vi "Discovery Loop Async.vi"(11 "DiscoveryService in":refnum<class "DiscoveryService.lvclass">) -> ()   [LabVIEW 2020, in "Vecto.lvlib" / "DiscoveryService.lvclass"]
uses:
  DiscoveryService.lvclass
  DiscoveryService.lvclass/DiscoveryService.ctl
  lv-volatus/messages/Discovery/Class/Msg.lvclass
  lv-volatus/messages/ServiceType/Enumeration.ctl
  lv-volatus/messages/ServiceType/ServiceType.lvlib
  lv-volatus/messages/Service/Data.ctl
  lv-volatus/messages/Service/Service.lvlib
  lv-volatus/messages/Discovery/Data.ctl
  lv-volatus/messages/Discovery/Discovery.lvlib
panel:
  out "Nodes":T1[](array[typedef])
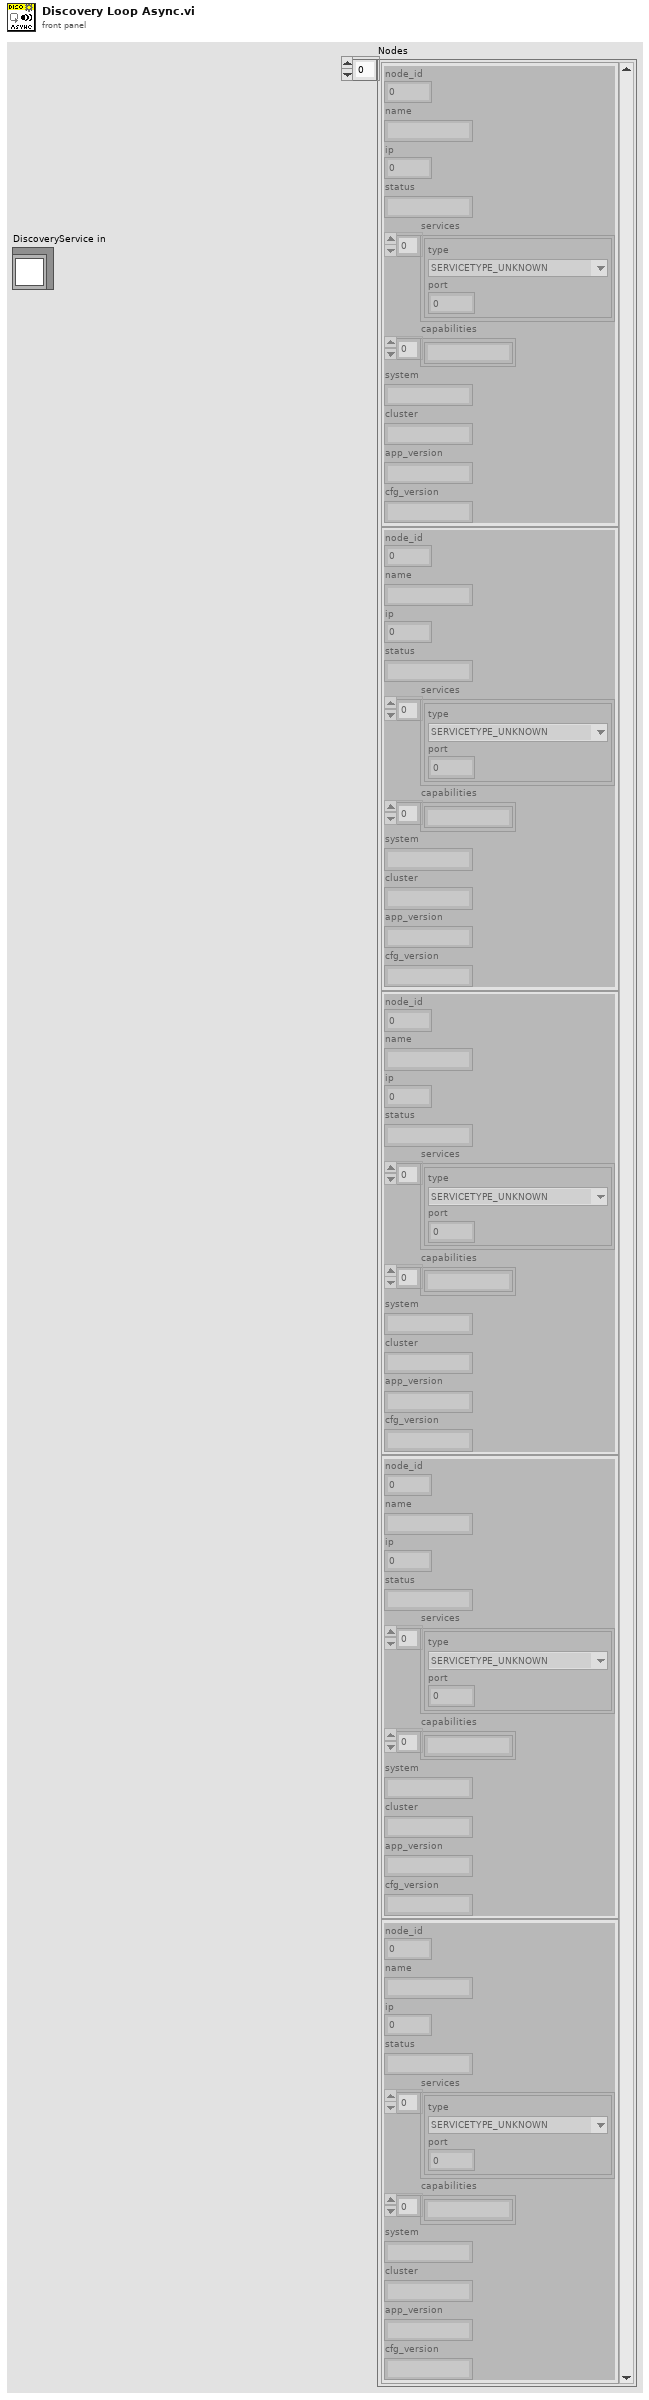
[diagram p1: front panel]
types:
  T1 = typedef "Discovery.lvlib/Data.ctl" = cluster{"node_id":u32, "name":string, "ip":u32, "status":string, "services":T2[], "capabilities":string[], "system":string, "cluster":string, "app_version":string, "cfg_version":string}
  T2 = typedef "Service.lvlib/Data.ctl" = cluster{"type":T3, "port":i32}
  T3 = typedef "ServiceType.lvlib/Enumeration.ctl" = enum16{"SERVICETYPE_UNKNOWN", "SERVICETYPE_TCPSERVER", "SERVICETYPE_HTTPSERVER"}
  T4 = typedef "Vecto.lvlib/DiscoveryService.lvclass/Capabilities Action.ctl" = enum16{"Add", "Remove", "Clear"}
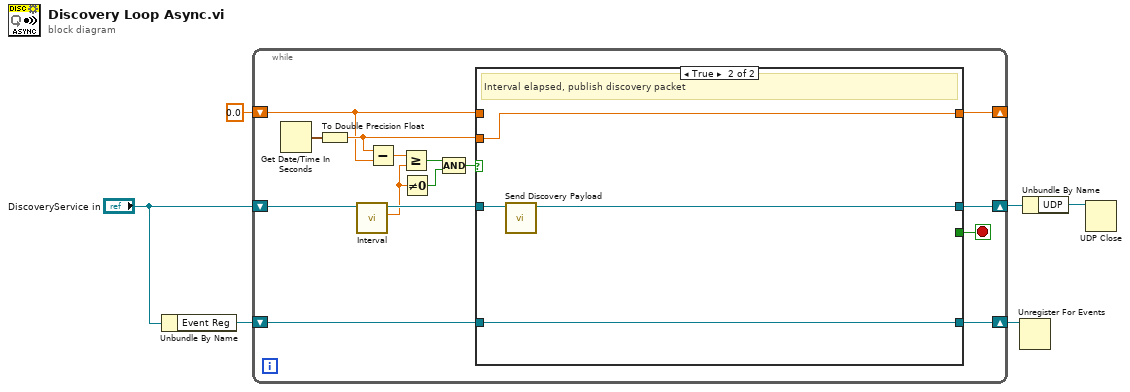
[diagram p0: block diagram]
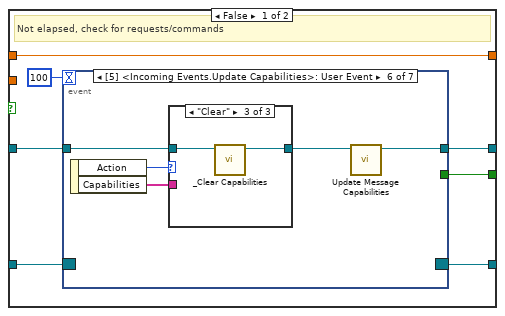
[diagram p2: hidden frame]
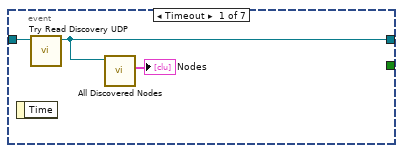
[diagram p3: hidden frame]
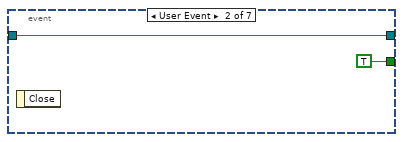
[diagram p4: hidden frame]
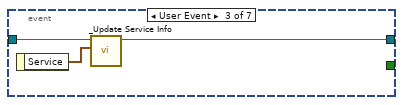
[diagram p5: hidden frame]
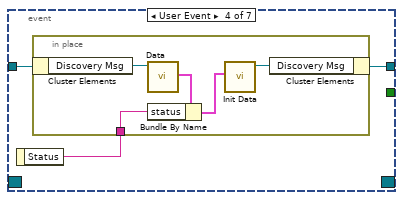
[diagram p6: hidden frame]
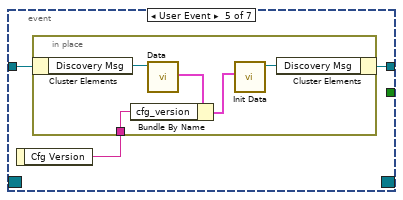
[diagram p7: hidden frame]
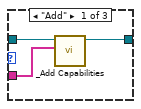
[diagram p8: hidden frame]
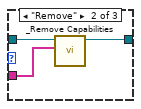
[diagram p9: hidden frame]
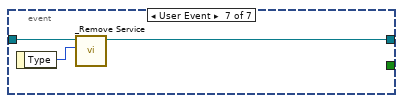
[diagram p10: hidden frame]
diagram:
  n1 = Unbundle By Name("DiscoveryService in") -> ("Event Reg"=w4:refnum<event-registration>)
  n2 = while {
    shift-right: [w15] -> _
    shift-left: 0.0 -> [w17]
    shift-right: [w14] -> w2
    shift-left: "DiscoveryService in" -> [w19]
    shift-right: [w12] -> w3
    shift-left: w4 -> [w13]
    stop <- w11 stop-if-true
    n3 = Get Date/Time In Seconds() -> (seconds since 1Jan1904=w21:timestamp)
    n4 = To Double Precision Float(number=w21) -> (double precision float=w18:dbl)
    n5 = call "Interval.vi"("DiscoveryService in"=w19) -> ("Interval S"=w8:dbl, "DiscoveryService out"=w10:refnum<class "DiscoveryService.lvclass">)  [unwired: 8 in, 1 out]
    n6 = Subtract(x=w18, y=w17) -> (x-y=w20:dbl)
    n7 = Greater Or Equal?(x=w20, y=w8) -> (x >= y?=w16:bool)
    n8 = Not Equal To 0?(x=w8) -> (x != 0?=w7:bool)
    n9 = Compound Arithmetic op=AND(w16, w7) -> (w9:bool)
    n10 = case shown="True" w9 {
      tunnel: w10 -> [w26 w71]
      tunnel: w18 -> [_ w72]
      tunnel: w17 -> [w28 _]
      tunnel: [w28 w72] -> w15
      tunnel: [w25 w70] -> w14
      tunnel: w13 -> [w24 w69]
      tunnel: [w23 w69] -> w12
      tunnel: [w22 _] -> w11
      frame False {
        # "Not elapsed, check for requests/commands"
        n11 = event shown="[5] <Incoming Events.Update Capabilities>: User Event" {
          selector: w24 -> [_ _ _ _ _ _ _]
          dyn-events: [_ _ _ _ _ _ _] -> w23
          timeout: 100 -> [_ _ _ _ _ _ _]
          tunnel: w26 -> [w31 w33 w36 w39 w47 w57 w68]
          tunnel: [w30 w33 w34 w37 w45 w53 w66] -> w25
          tunnel: [_ TRUE _ _ _ _ _] -> w22
          event Timeout {
            n12 = event-data() -> ()  [unwired: 1 in, 1 out]
            n13 = call "Try Read Discovery UDP.vi"("DiscoveryService in"=w31) -> ("DiscoveryService out"=w30:refnum<class "DiscoveryService.lvclass">)  [unwired: 9 in, 1 out]
            n14 = call "All Discovered Nodes.vi"("DiscoveryService in"=w30) -> ("Nodes"=→"Nodes":T1[])  [unwired: 8 in, 2 out]
          }
          event User Event {
            n15 = event-data() -> ()  [unwired: 1 in, 1 out]
          }
          event User Event {
            n16 = event-data() -> ("Service"=w35:T2)  [unwired: 1 in]
            n17 = call "_Update Service Info.vi"("Service"=w35, "DiscoveryService in"=w36) -> ("DiscoveryService out"=w34:refnum<class "DiscoveryService.lvclass">)  [unwired: 8 in, 1 out]
          }
          event User Event {
            n18 = event-data() -> ("Status"=w38:string)  [unwired: 1 in]
            n19 = in-place {
              in-place-border: w38 -> [w42]
              n20 = in-place-cluster #1(w39) -> ("Discovery Msg"=w44:refnum<class "Msg.lvclass">)
              n21 = call "Data.vi"("PB Msg Template in"=w44) -> ("Data"=w43:T1)  [unwired: 8 in, 2 out]
              n22 = Bundle By Name(cluster=w43, "status"=w42) -> (w41:T1)
              n23 = call "Init Data.vi"("Data"=w41) -> ("Msg out"=w40:refnum<class "Msg.lvclass">)  [unwired: 10 in]
              n24 = in-place-cluster #1("Discovery Msg"=w40) -> (w37:refnum<class "DiscoveryService.lvclass">)
            }
          }
          event User Event {
            n25 = event-data() -> ("Cfg Version"=w46:string)  [unwired: 1 in]
            n26 = in-place {
              in-place-border: w46 -> [w50]
              n27 = in-place-cluster #2(w47) -> ("Discovery Msg"=w52:refnum<class "Msg.lvclass">)
              n28 = call "Data.vi"("PB Msg Template in"=w52) -> ("Data"=w51:T1)  [unwired: 8 in, 2 out]
              n29 = Bundle By Name(cluster=w51, "cfg_version"=w50) -> (w49:T1)
              n30 = call "Init Data.vi"("Data"=w49) -> ("Msg out"=w48:refnum<class "Msg.lvclass">)  [unwired: 10 in]
              n31 = in-place-cluster #2("Discovery Msg"=w48) -> (w45:refnum<class "DiscoveryService.lvclass">)
            }
          }
          event User Event {
            n32 = event-data() -> ("Action"=w55:T4, "Capabilities"=w54:string[])  [unwired: 1 in]
            n33 = case shown="\"Clear\"" w55 {
              tunnel: w57 -> [w60 w63 w65]
              tunnel: [w59 w62 w64] -> w56
              tunnel: w54 -> [w58 w61 _]
              frame "Add" {
                n34 = call "_Add Capabilities.vi"("Capabilities"=w58, "NodeDiscovery in"=w60) -> ("NodeDiscovery out"=w59:refnum<class "DiscoveryService.lvclass">)  [unwired: 8 in, 1 out]
              }
              frame "Remove" {
                n35 = call "_Remove Capabilities.vi"("Capabilities"=w61, "NodeDiscovery in"=w63) -> ("NodeDiscovery out"=w62:refnum<class "DiscoveryService.lvclass">)  [unwired: 8 in, 1 out]
              }
              frame "Clear" {
                n36 = call "_Clear Capabilities.vi"("NodeDiscovery in"=w65) -> ("NodeDiscovery out"=w64:refnum<class "DiscoveryService.lvclass">)  [unwired: 9 in, 1 out]
              }
            }
            n37 = call "Update Message Capabilities.vi"("NodeDiscovery in"=w56) -> ("NodeDiscovery out"=w53:refnum<class "DiscoveryService.lvclass">)  [unwired: 9 in, 1 out]
          }
          event User Event {
            n38 = event-data() -> ("Type"=w67:T3)  [unwired: 1 in]
            n39 = call "_Remove Service.vi"("Type"=w67, "DiscoveryService in"=w68) -> ("DiscoveryService out"=w66:refnum<class "DiscoveryService.lvclass">)  [unwired: 8 in, 1 out]
          }
        }
      }
      frame True {
        # "Interval elapsed, publish discovery packet"
        n40 = call "Send Discovery Payload.vi"("DiscoveryService in"=w71) -> ("DiscoveryService out"=w70:refnum<class "DiscoveryService.lvclass">)  [unwired: 9 in, 1 out]
      }
    }
  }
  n41 = Unregister For Events(event registration refnum=w3) -> ()  [unwired: 1 in, 1 out]
  n42 = Unbundle By Name(w2) -> ("UDP"=w1:refnum<k16>)
  n43 = UDP Close(connection ID=w1) -> ()  [unwired: 1 in, 2 out]
